vi "Write SPI Bus.vi"(8 "error in (no error)":errorcluster, 10 "SPI Bus":T1=enum."Invalid", 11 "navX - SPI in":refnum<class "navX - SPI.lvclass">) -> (0 "error out":errorcluster, 3 "navX - SPI out":refnum<class "navX - SPI.lvclass">)   [LabVIEW 2015, in "navX Library v3.lvlib" / "navX - SPI.lvclass"]
uses:
  navX - SPI.lvclass
  <vilib>/Rock Robotics/SystemInterfaces/spilib/spi_bus.ctl
  navX - SPI.lvclass/navX - SPI.ctl
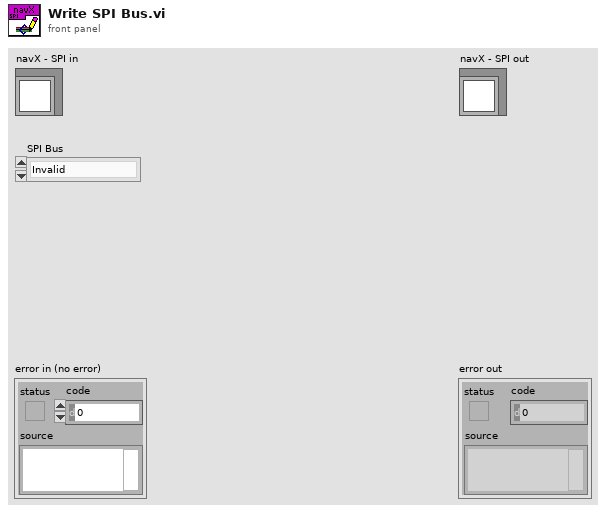
[diagram p1: front panel]
types:
  T1 = typedef "spi_bus.ctl" = enum16{"SPI On-Board, CS0", "SPI On-Board, CS1", "SPI On-Board, CS2", "SPI On-Board, CS3", "SPI MXP", "Invalid"}
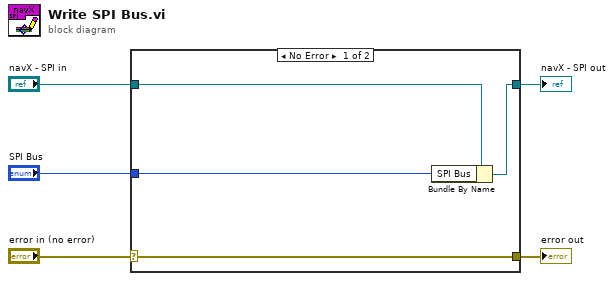
[diagram p0: block diagram]
diagram:
  n1 = case shown="No Error" "error in (no error)" {
    selector: "error in (no error)" -> [w9 w10]
    tunnel: [w9 w10] -> w4
    tunnel: [w7 w11] -> w2
    tunnel: "navX - SPI in" -> [w8 w11]
    tunnel: "SPI Bus" -> [w6 _]
    frame No Error {
      n2 = Bundle By Name(cluster=w8, "SPI Bus"=w6) -> (w7:refnum<class "navX - SPI.lvclass">)
    }
    frame Error {
    }
  }
  "error out" <- w4
  "navX - SPI out" <- w2
